vi "_Fit VI window to Largest Dec.vi"(4 "error in (no error)":errorcluster, 6 "border spacing (2 px)":i32=2, 7 "VI Ref (calling VI)":refnum<vi>) -> (0 "error out":errorcluster, 3 "dup VI Ref":refnum<vi>)   [LabVIEW 2017]
doc: "This utility will fit (resize and center) a VI (defined by the \"VI Ref\" input) about the largest decoration in that VI. It will add a border defined by border spacing in units of pixels. If there are no decorations found in the VI it is a no-op and will not produce an error. Unfortunately, this VI can not find locked decorations (yet)."
panel:
  # "Fit VI window to Largest Decoration.vi\n\nFits a VI's front panel window to its largest decoration size.\n\nPlease visit http://www.OpenG.org to learn about the\nOpen Source LabVIEW software movement.\n\nNOTICE -- YOU MUST LEAVE THIS NOTICE IN PLACE.  PER THE TERMS OF THE LICENSE BELOW, YOU MAY SUBLICENSE THIS SOFTWARE \nIN ANY WAY THAT DOES NOT CONFLICT WITH THIS LICENSE.\n\n### BSD License (http://www.opensource.org/licenses/bsd-license.php) Begin ###\n \nCopyright (c) 2002, Jim Kring <jim@jimkring.com>\nCopyright (c) 2002, Cal-Bay Systems, Inc. <info@calbay.com>\n\nAll rights reserved.\n\nRedistribution and use in source and binary forms, with or without modification, are permitted provided that the following conditions are met:\n\n    * Redistributions of source code must retain the above copyright notice, this list of conditions and the following disclaimer.\n    * Redistributions in binary form must reproduce the above copyright notice, this list of conditions and the following disclaimer in the \n       documentation and/or other materials provided with the distribution.\n    * Neither the name of SciWare, James Kring, Inc., nor the names of its contributors may be used to endorse or promote products derived \n       from this software without specific prior written permission.\n\nTHIS SOFTWARE IS PROVIDED BY THE COPYRIGHT HOLDERS AND CONTRIBUTORS \"AS IS\" AND ANY EXPRESS OR IMPLIED WARRANTIES, \nINCLUDING, BUT NOT LIMITED TO, THE IMPLIED WARRANTIES OF MERCHANTABILITY AND FITNESS FOR A PARTICULAR PURPOSE ARE \nDISCLAIMED. IN NO EVENT SHALL THE COPYRIGHT OWNER OR CONTRIBUTORS BE LIABLE FOR ANY DIRECT, INDIRECT, INCIDENTAL,\n SPECIAL, EXEMPLARY, OR CONSEQUENTIAL DAMAGES (INCLUDING, BUT NOT LIMITED TO, PROCUREMENT OF SUBSTITUTE GOODS OR \nSERVICES; LOSS OF USE, DATA, OR PROFITS; OR BUSINESS INTERRUPTION) HOWEVER CAUSED AND ON ANY THEORY OF LIABILITY, \nWHETHER IN CONTRACT, STRICT LIABILITY, OR TORT (INCLUDING NEGLIGENCE OR OTHERWISE) ARISING IN ANY WAY OUT OF THE USE \nOF THIS SOFTWARE, EVEN IF ADVISED OF THE POSSIBILITY OF SUCH DAMAGE.\n\n### BSD License End ###"
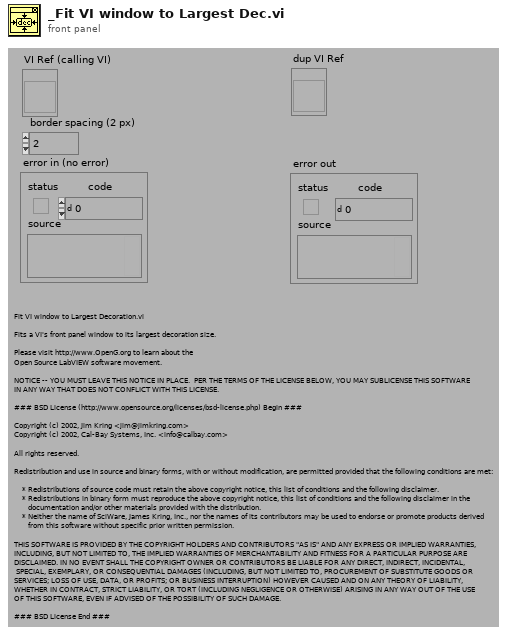
[diagram p1: front panel]
types:
  T1 = typedef "LVRectTypeDef.ctl" = cluster{"Left":i16, "Top":i16, "Right":i16, "Bottom":i16}
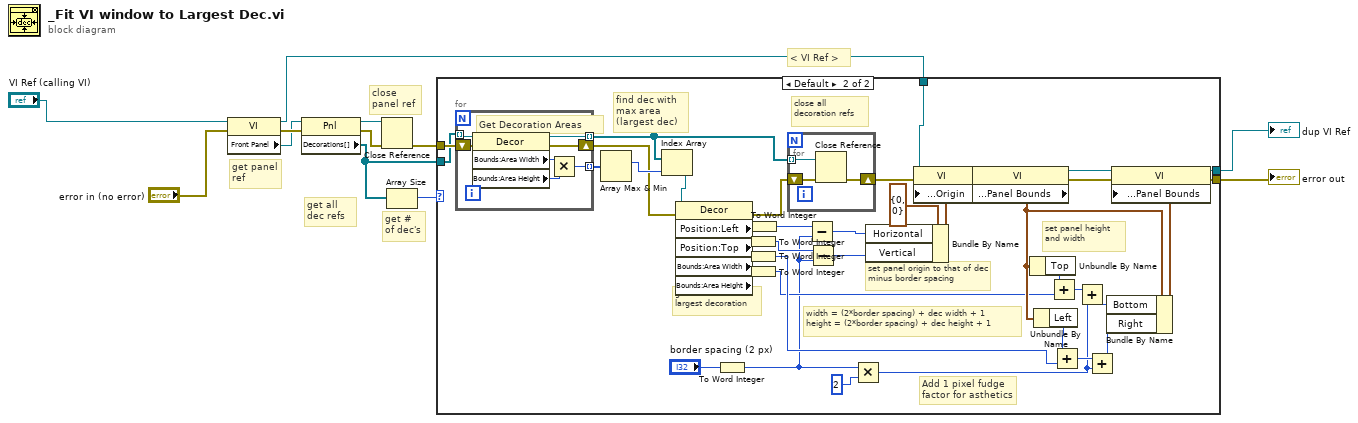
[diagram p0: block diagram]
diagram:
  # "get # of dec's"
  # "get panel ref"
  # "get all dec refs"
  # "close panel ref"
  # "< VI Ref >"
  n1 = property on="Property Node" class="VI"(reference="VI Ref (calling VI)", error in="error in (no error)") -> (reference out=w12:refnum<vi>, error out=w10:errorcluster, "Front Panel"=w7:refnum<vi>)
  n2 = property on="Property Node" class="Pnl"(reference=w7, error in=w10) -> (reference out=w11:refnum<vi>, error out=w9:errorcluster, "Decorations[]"=w4:refnum<vi>[])
  n3 = Close Reference(reference=w11, error in (no error)=w9) -> (error out=w6:errorcluster)
  n4 = Array Size(array=w4) -> (size(s)=w3:i32)
  n5 = case shown="Default" w3 {
    tunnel: w12 -> [w14 w52]
    tunnel: w6 -> [w13 w35]
    tunnel: [w13 w23] -> w5
    tunnel: [w14 w22] -> w1
    tunnel: w4 -> [_ w21]
    frame 0 {
      # "do nothing if no decorations"
    }
    frame Default {
      # "width = (2*border spacing) + dec width + 1\nheight = (2*border spacing) + dec height + 1"
      # "set panel height and width"
      # "set panel origin to that of dec minus border spacing"
      # "close all  decoration refs"
      # "get coord's of largest decoration"
      # "Add 1 pixel fudge factor for asthetics"
      # "find dec with max area (largest dec)"
      n6 = for {
        tunnel: w21 -> [w61] mode=indexing
        tunnel: [w58] -> w34 mode=indexing
        shift-right: [w56] -> w30
        shift-left: w35 -> [w57]
        tunnel: [w55] -> w32 mode=indexing
        # "Get Decoration Areas"
        n7 = property class="Decor"(reference=w61, error in=w57) -> (reference out=w55:refnum<vi>, error out=w56:errorcluster, "Bounds:Area Width"=w60:u32, "Bounds:Area Height"=w59:u32)
        n8 = Multiply(x=w60, y=w59) -> (x*y=w58:u32)
      }
      n9 = Array Max & Min(array=w34) -> (max index (indices)=w33:i32)  [unwired: 3 out]
      n10 = Index Array(array=w32, index=w33) -> (element=w31:refnum<vi>)
      n11 = property class="Decor"(reference=w31, error in=w30) -> (error out=w29:errorcluster, "Position:Left"=w38:i32, "Position:Top"=w41:i32, "Bounds:Area Width"=w46:u32, "Bounds:Area Height"=w44:u32)  [unwired: 1 out]
      n12 = To Word Integer(number="border spacing (2 px)") -> (16bit integer=w15:i16)
      n13 = To Word Integer(number=w41) -> (16bit integer=w16:i16)
      n14 = To Word Integer(number=w46) -> (16bit integer=w19:i16)
      n15 = To Word Integer(number=w44) -> (16bit integer=w18:i16)
      n16 = To Word Integer(number=w38) -> (16bit integer=w17:i16)
      n17 = for {
        tunnel: w32 -> [w64] mode=indexing
        shift-right: [w62] -> w26
        shift-left: w29 -> [w63]
        n18 = Close Reference(reference=w64, error in (no error)=w63) -> (error out=w62:errorcluster)
      }
      n19 = Subtract(x=w17, y=w15) -> (x-y=w39:i16)
      n20 = Subtract(x=w16, y=w15) -> (x-y=w40:i16)
      n21 = Multiply(x=w15, y=i16 2) -> (x*y=w20:i16)
      n22 = Bundle By Name(cluster=cluster{"Horizontal":i16, "Vertical":i16} {"Horizontal"=0, "Vertical"=0} ("Front Panel Window:Origin"), "Horizontal"=w39, "Vertical"=w40) -> (w36:cluster{"Horizontal":i16, "Vertical":i16})
      n23 = property on="Property Node" class="VI"(reference=w52, error in=w26, "Front Panel Window:Origin"=w36) -> (reference out=w53:refnum<vi>, error out=w25:errorcluster)
      n24 = property on="Property Node" class="VI"(reference=w53, error in=w25) -> (reference out=w54:refnum<vi>, error out=w24:errorcluster, "Front Panel Window:Panel Bounds"=w42:T1)
      n25 = Unbundle By Name(w42) -> ("Top"=w43:i16)
      n26 = Unbundle By Name(w42) -> ("Left"=w45:i16)
      n27 = Add(x=w43, y=w18) -> (x+y=w50:i16)
      n28 = Add(x=w45, y=w19) -> (x+y=w48:i16)
      n29 = Add(x=w50, y=w20) -> (x+y=w51:i16)
      n30 = Add(x=w48, y=w20) -> (x+y=w49:i16)
      n31 = Bundle By Name(cluster=w42, "Bottom"=w51, "Right"=w49) -> (w47:T1)
      n32 = property on="Property Node" class="VI"(reference=w54, error in=w24, "Front Panel Window:Panel Bounds"=w47) -> (reference out=w22:refnum<vi>, error out=w23:errorcluster)
    }
  }
  "error out" <- w5
  "dup VI Ref" <- w1
